vi "FTW-Collection-GetAllValues.vi"(0 "Collection":refnum<class "FTW-Collection.lvclass">, 11 "error in":errorcluster) -> (4 "Collection out":refnum<class "FTW-Collection.lvclass">, 6 "Key-Variant Pairs":T1[](array[typedef]), 15 "error out":errorcluster)   [LabVIEW 2012, in "FTW-Collection.lvclass"]
uses:
  FTW-Collection.lvclass
  FTW-Collection-KeyVariantPair.ctl
  FTW-Collection.lvclass/FTW-Collection.ctl
panel:
  # "Inputs"
  # "Outputs"
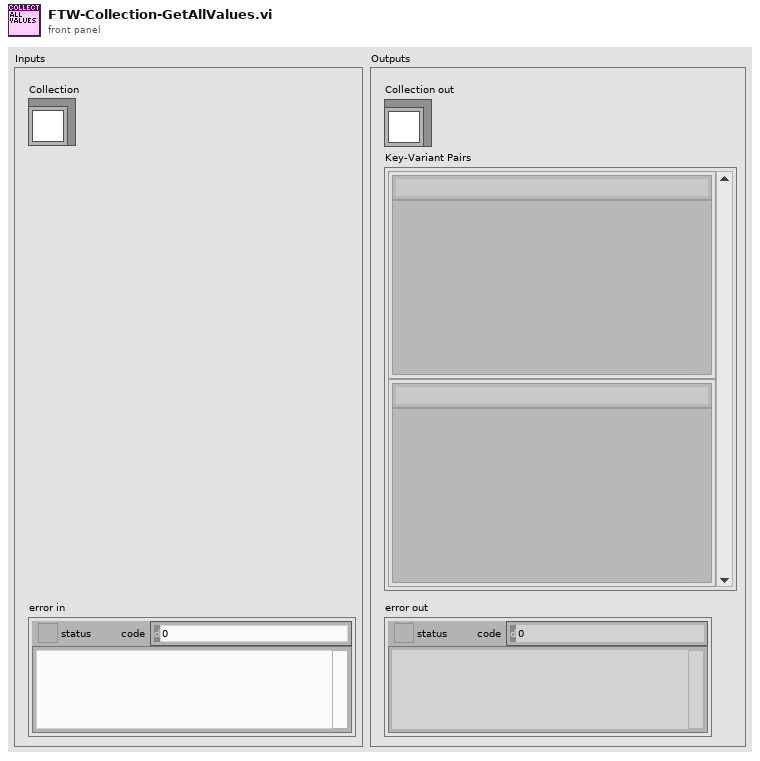
[diagram p1: front panel]
types:
  T1 = typedef "FTW-Collection-KeyVariantPair.ctl" = cluster{"Key":string, "Value":variant}
  T2 = cluster{"Unescaped JSON String":string, variant}[]
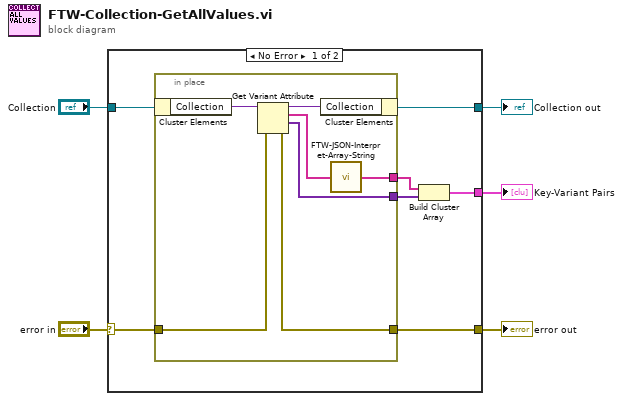
[diagram p0: block diagram]
diagram:
  n1 = case shown="No Error" "error in" {
    selector: "error in" -> [w10 w21]
    tunnel: [w9 w21] -> w5
    tunnel: [w11 w20] -> w3
    tunnel: "Collection" -> [w12 w20]
    tunnel: [w6 _] -> w1
    frame No Error {
      n2 = in-place {
        in-place-border: w10 -> [w19]
        in-place-border: [w18] -> w9
        in-place-border: [w13] -> w8
        in-place-border: [w15] -> w7
        n3 = in-place-cluster #1(w12) -> ("Collection"=w17:variant)
        n4 = Get Variant Attribute(Variant=w17, error in=w19) -> (duplicate Variant=w16:variant, names=w14:string[], values=w15:variant[], error out=w18:errorcluster)  [unwired: 2 in]
        n5 = in-place-cluster #1("Collection"=w16) -> (w11:refnum<class "FTW-Collection.lvclass">)
        n6 = call "FTW-JSON-Interpret-Array-String.vi"("Escaped JSON Strings"=w14) -> ("LabVIEW Strings"=w13:string[])
      }
      n7 = Build Cluster Array(w8, w7) -> (w6:T2)
    }
    frame Error {
    }
  }
  "error out" <- w5
  "Collection out" <- w3
  "Key-Variant Pairs" <- w1
